vi "User Event LV2-Receive.vi"(0 "Event Name":string, 5 "Data":variant, 11 "Error In":errorcluster, 13 "Operation":T1) -> (4 "User Event Ref":refnum<user-event>, 15 "Error Out":errorcluster)   [LabVIEW 2023]
doc: "The file is the Functional global to store the user event reference to transmit data."
uses:
  Controls/User Event Operations.ctl
  Controls/Queue Element.ctl
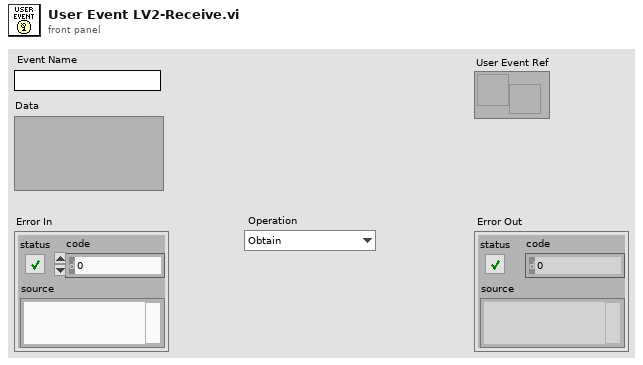
[diagram p1: front panel]
types:
  T1 = typedef "User Event Operations.ctl" = enum16{"Obtain", "Generate", "Destroy"}
  T2 = typedef "Queue Element.ctl" = cluster{"State":string, "Data":variant}
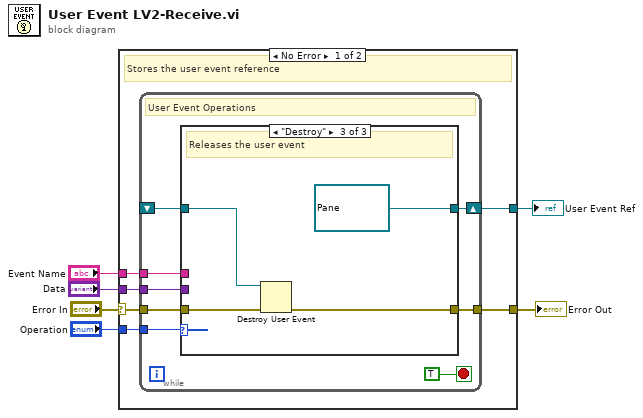
[diagram p0: block diagram]
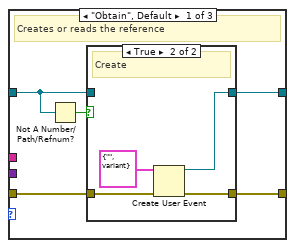
[diagram p2: hidden frame]
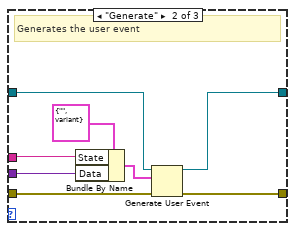
[diagram p4: hidden frame]
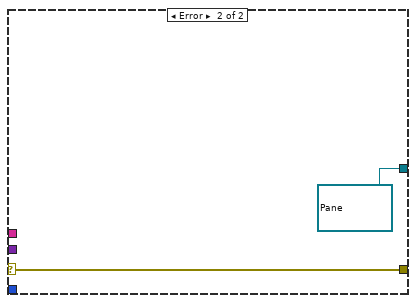
[diagram p5: hidden frame]
diagram:
  n1 = case shown="No Error" "Error In" {
    selector: "Error In" -> [w11 w45]
    tunnel: "Operation" -> [w12 _]
    tunnel: [w10 w45] -> w4
    tunnel: [w7 refnum<user-event> refnum ("User Event Data")] -> w3
    tunnel: "Data" -> [w9 _]
    tunnel: "Event Name" -> [w8 _]
    frame No Error {
      # "Stores the user event reference"
      n2 = while {
        tunnel: w12 -> [w20]
        tunnel: w11 -> [w19]
        tunnel: [w18] -> w10
        shift-right: [w17] -> w7
        shift-left: _ -> [w16]
        tunnel: w9 -> [w14]
        tunnel: w8 -> [w13]
        stop <- TRUE stop-if-true
        # "User Event Operations"
        n3 = case shown="\"Destroy\"" w20 {
          tunnel: w19 -> [w24 w39 w42]
          tunnel: [w25 w38 w43] -> w18
          tunnel: [w23 w36 refnum<user-event> refnum ("User Event Data")] -> w17
          tunnel: w16 -> [w22 w37 w41]
          tunnel: w14 -> [_ w35 _]
          tunnel: w13 -> [_ w34 _]
          frame "Obtain", Default {
            # "Creates or reads the reference"
            n4 = Not A Number/Path/Refnum?(number/path/refnum=w22) -> (NaN/Path/Refnum?=w21:bool)
            n5 = case shown="True" w21 {
              tunnel: [w26 w31] -> w25
              tunnel: w24 -> [w26 w30]
              tunnel: [w27 w29] -> w23
              tunnel: w22 -> [w27 _]
              frame False {
                # "Use existing"
              }
              frame True {
                # "Create"
                n6 = Create User Event(user event datatype=T2 {"State"="", "Data"=variant} ("User Event Data"), error in=w30) -> (user event=w29:refnum<user-event>, error out=w31:errorcluster)
              }
            }
          }
          frame "Generate" {
            # "Generates the user event"
            n7 = Bundle By Name(cluster=T2 {"State"="", "Data"=variant} ("User Event Data"), "State"=w34, "Data"=w35) -> (w33:T2)
            n8 = Generate User Event(user event=w37, event data cluster=w33, error in=w39) -> (user event out=w36:refnum<user-event>, error out=w38:errorcluster)  [unwired: 1 in]
          }
          frame "Destroy" {
            # "Releases the user event"
            n9 = Destroy User Event(user event=w41, error in=w42) -> (error out=w43:errorcluster)
          }
        }
      }
    }
    frame Error {
    }
  }
  "Error Out" <- w4
  "User Event Ref" <- w3
